vi "Peak Detector no State.vi"(0 "X":dbl[](array[numeric]) format="%0.2f", 1 "end of data (T)":bool=TRUE, 2 "initialize (T)":bool=TRUE, 5 "threshold":dbl format="%0.2f", 7 "width":i32=3 min=3, 9 "peaks/valleys":enum32{"Peaks", "Valleys"}(ring), 11 "error in":errorcluster, 12 "state info":T1) -> (3 "# found":i32, 4 "Locations":dbl[](array[numeric]) format="%0.2f", 6 "Amplitudes":dbl[](array[numeric]) format="%0.2f", 8 "2nd Derivatives":dbl[](array[numeric]) format="%0.2f", 14 "state info":T1, 15 "error out":errorcluster)   [LabVIEW 2020, in "NI_MAPro.lvlib"]
doc: "Finds the location, amplitude, and second derivative of peaks or valleys in the input signal."
uses:
  NI_MAPro.lvlib
  NI_MABase.lvlib
  <resource>/lvanlys.dll
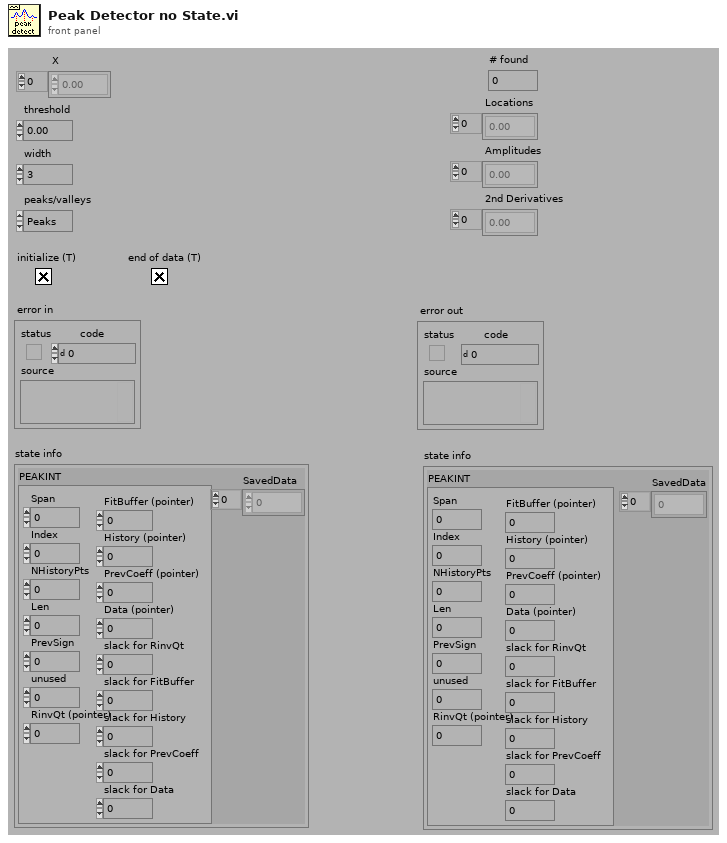
[diagram p1: front panel]
types:
  T1 = cluster{"PEAKINT":cluster{"Span":i32, "Index":i32, "NHistoryPts":i32, "Len":i32, "PrevSign":i32, "unused":i32, "RinvQt (pointer)":u32, "FitBuffer (pointer)":u32, "History (pointer)":u32, "PrevCoeff (pointer)":u32, "Data (pointer)":u32, "slack for RinvQt":u32, "slack for FitBuffer":u32, "slack for History":u32, "slack for PrevCoeff":u32, "slack for Data":u32}, "SavedData":dbl[]}
  T2 = cluster{"Span":i32, "Index":i32, "NHistoryPts":i32, "Len":i32, "PrevSign":i32, "unused":i32, "RinvQt (pointer)":u32, "FitBuffer (pointer)":u32, "History (pointer)":u32, "PrevCoeff (pointer)":u32, "Data (pointer)":u32, "slack for RinvQt":u32, "slack for FitBuffer":u32, "slack for History":u32, "slack for PrevCoeff":u32, "slack for Data":u32}
  T3 = cluster{"X":dbl[], "threshold":dbl, "upper limit":i32, "peaks/valleys":enum32{"Peaks", "Valleys"}, "Array Constant":dbl[], "Array Constant":dbl[], "Array Constant":dbl[], i32, i32}
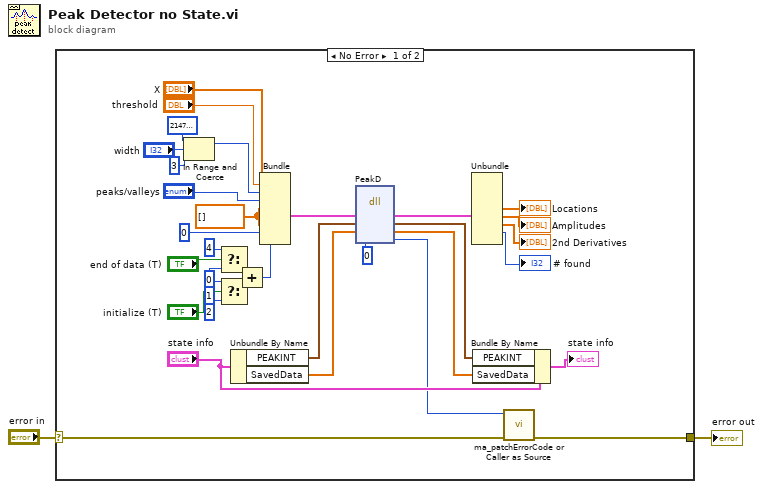
[diagram p0: block diagram]
diagram:
  n1 = case shown="No Error" "error in" {
    selector: "error in" -> [w8 w37]
    tunnel: [w7 w37] -> w1
    frame No Error {
      w16 = dbl[] [] ("Array Constant")
      n2 = In Range and Coerce(upper limit=2147483647, x="width", lower limit=3) -> (coerced(x)=w4:i32)  [unwired: 1 out]
      n3 = Select(t=4, s="end of data (T)", f=0) -> (s? t:f=w34:i32)
      n4 = Select(t=1, s="initialize (T)", f=2) -> (s? t:f=w35:i32)
      n5 = Unbundle By Name("state info") -> ("PEAKINT"=w15:T2, "SavedData"=w10:dbl[])
      n6 = Add(x=w34, y=w35) -> (x+y=w25:i32)
      n7 = Bundle("X"="X", "threshold"="threshold", "upper limit"=w4, "peaks/valleys"="peaks/valleys", "Array Constant"=w16, "Array Constant"=w16, "Array Constant"=w16, 0, w25) -> (w23:T3)  [unwired: 1 out]
      n8 = dll-call lib="C:/Program Files (x86)/National Instruments/LabVIEW 2020/resource/lvanlys.*" fn="PeakD"("PeakApp"=w23, "pPEAKINT"=w15, "SavedData"=w10, "pErr"=0) -> ("PeakApp"=w22:T3, "pPEAKINT"=w14:T2, "SavedData"=w13:dbl[], "pErr"=w9:i32)  [unwired: 3 in, 3 out]
      n9 = Unbundle(w22) -> ("Array Constant"=→"Locations":dbl[], "Array Constant"=→"Amplitudes":dbl[], "Array Constant"=→"2nd Derivatives":dbl[], →"# found":i32)  [unwired: 5 out]
      n10 = Bundle By Name(cluster="state info", "PEAKINT"=w14, "SavedData"=w13) -> (→"state info":T1)
      n11 = call "ma_patchErrorCode or Caller as Source.vi"("error in (no error)"=w8, "error code"=w9) -> ("error out"=w7:errorcluster)  [unwired: 2 in, 7 out]
    }
    frame Error {
    }
  }
  "error out" <- w1
